vi "Create local tables from Server DB (old).vi"(8 "error in":errorcluster, 10 "Site":string="ICE1", 11 "tableNames":string[](array[string])) -> (0 "error out":errorcluster)   [LabVIEW 2010]
uses:
  <vilib>/addons/database/Auxilliary.llb/DB Tools DataTypes.ctl
  <vilib>/addons/database/Auxilliary.llb/DB Tools Cursor Type.ctl
  <vilib>/addons/database/_DB Variant To Data/Database Variant To Data.xnode
  <vilib>/addons/database/Connection.llb/DB Tools Open Connec (Path).vi
  <vilib>/addons/database/Connection.llb/Conn Execute.vi
  <vilib>/addons/database/Recordset.llb/Rec Fetch Recordset Data (R).vi
  <vilib>/addons/database/Recordset.llb/Rec Destroy - Connection.vi
  <vilib>/addons/database/NI_Database_API.lvlib
panel:
  out "column information":T2(array[cluster])
  out "columns":string[](array[string])
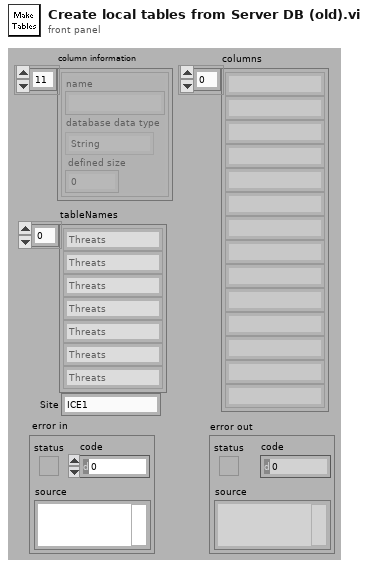
[diagram p1: front panel]
types:
  T1 = typedef "NI_Database_API.lvlib/DB Tools DataTypes.ctl" = enum16{"String", "Long (I32)", "Single (SGL)", "Double (DBL)", "Date/Time", "Binary"}
  T2 = cluster{"name":string, "database data type":T1, "defined size":i32}[]
  T3 = typedef "NI_Database_API.lvlib/DB Tools Cursor Type.ctl" = enum16{"forward-only", "keyset", "dynamic", "static"}
  T4 = typedef "NI_Database_API.lvlib/Conn ObjectReference.ctl" = refnum<k1>
  T5 = typedef "NI_Database_API.lvlib/Rec ObjectReference.ctl" = refnum<k1>
  T6 = cluster{"data":i32, "data":i32, "data":i32, "trimmed string":string, "trimmed string":string, "data":i32, "data":sgl, "data":i32, "data":i32, "data":i32, "trimmed string":string}
  T7 = cluster{"data":i32, "data":i32, "data":i32, "trimmed string":string, "data":i32, "data":i32, "trimmed string":string, "trimmed string":string, "trimmed string":string, "data":i32, "data":i32, "data":sgl, "data":i32, "data":i32, "trimmed string":string, "trimmed string":string}
  T8 = cluster{"data":i32, "trimmed string":string, "data":i32, "data":i32}
  T9 = cluster{"data":i32, "trimmed string":string, "data":i32, "trimmed string":string, "trimmed string":string, "trimmed string":string, "trimmed string":string, "data":sgl, "data":string, "trimmed string":string, "data":i32, "trimmed string":string, "trimmed string":string, "trimmed string":string}
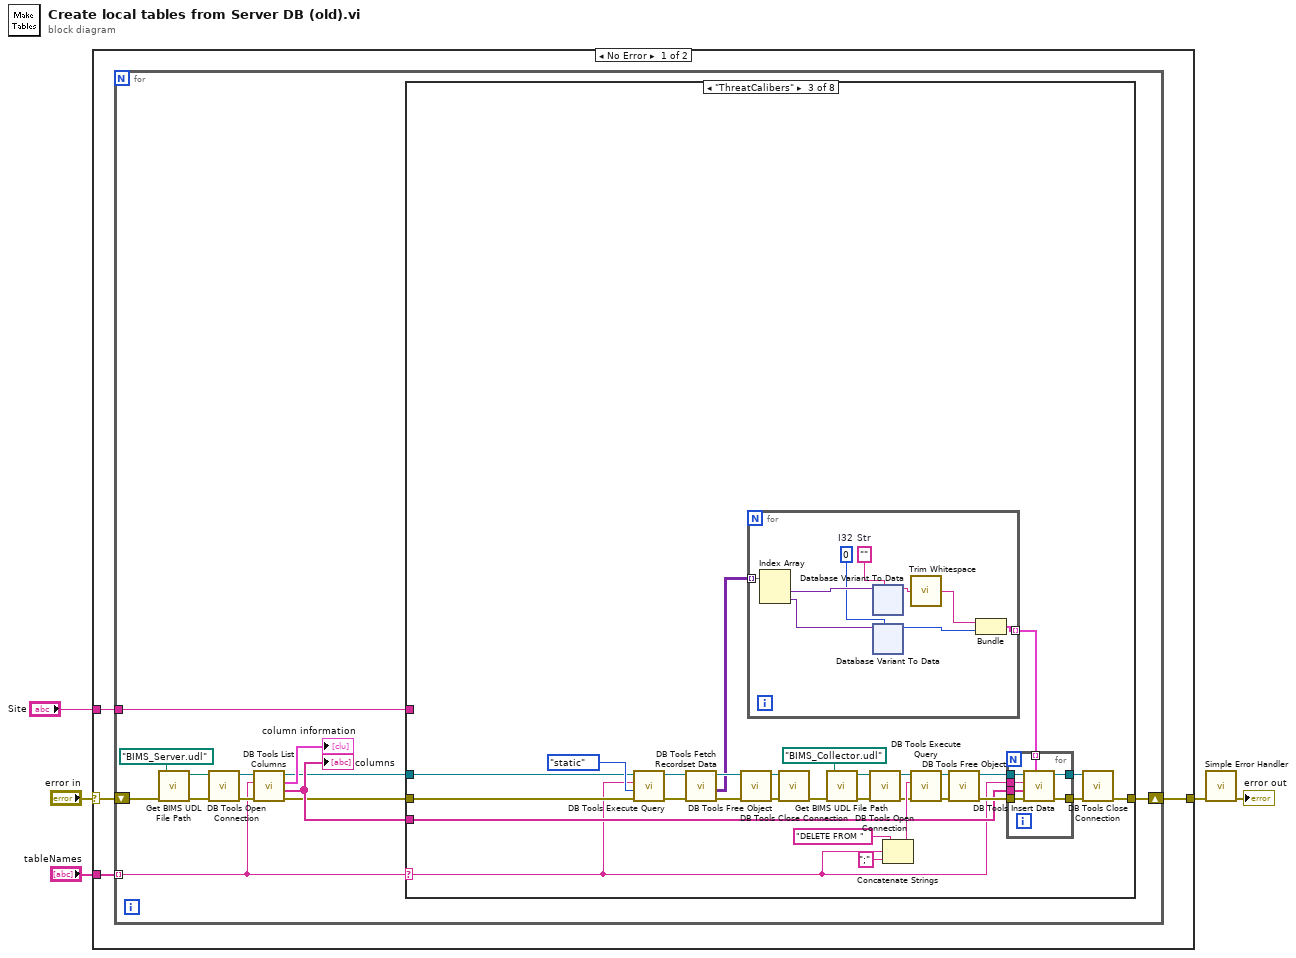
[diagram p0: block diagram]
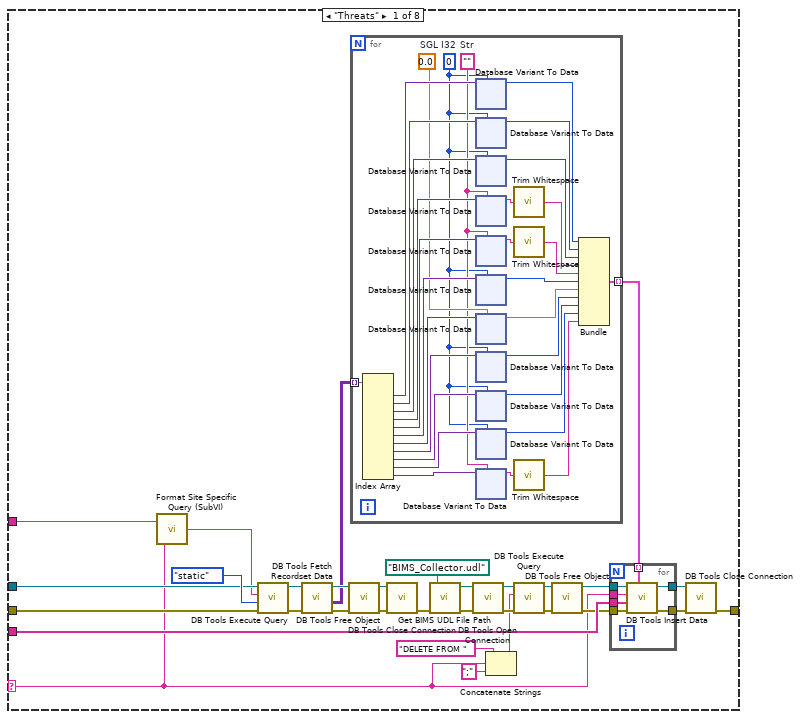
[diagram p2: hidden frame]
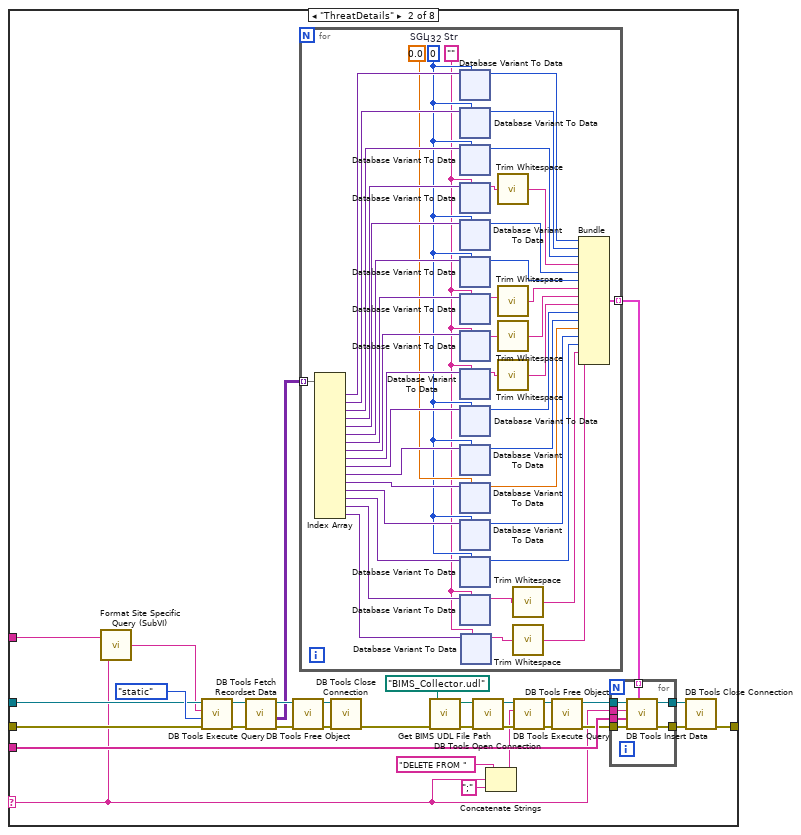
[diagram p3: hidden frame]
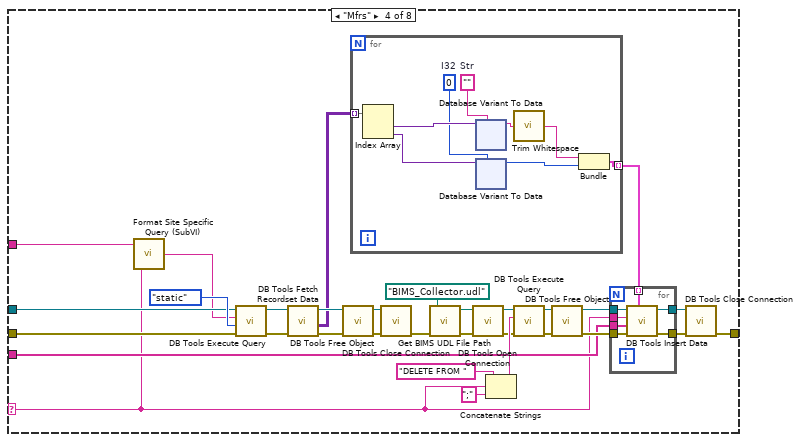
[diagram p4: hidden frame]
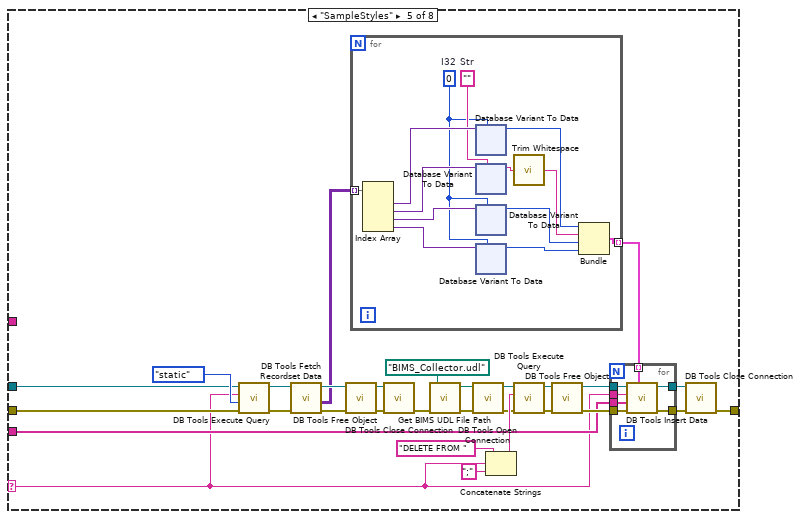
[diagram p5: hidden frame]
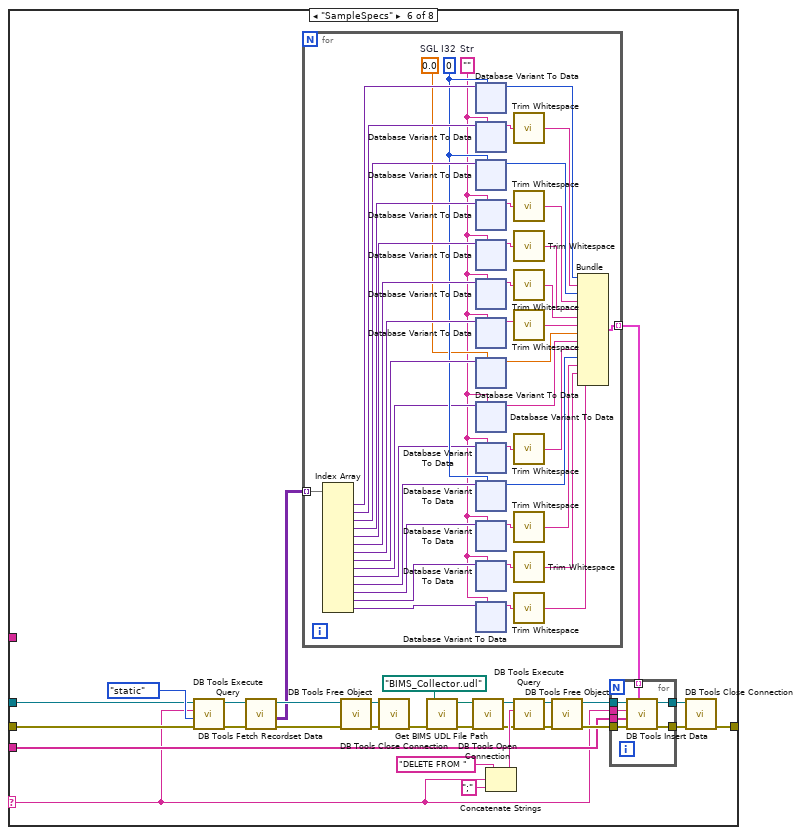
[diagram p6: hidden frame]
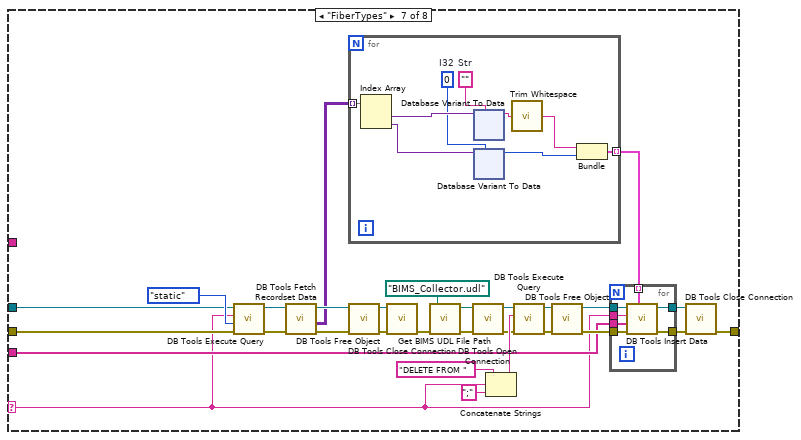
[diagram p7: hidden frame]
diagram:
  n1 = case shown="No Error" "error in" {
    selector: "error in" -> [w8 w2069]
    tunnel: [w9 w2069] -> w3
    tunnel: "tableNames" -> [w7 _]
    tunnel: "Site" -> [w6 _]
    frame No Error {
      n2 = for {
        tunnel: w7 -> [w16] mode=indexing
        shift-right: [w17] -> w9
        shift-left: w8 -> [w13]
        tunnel: w6 -> [w14]
        n3 = call "Get BIMS UDL File Path.vi"("error in"=w13, "UDL file name"=path "BIMS_Server.udl") -> ("error out"=w12:errorcluster, "Full UDL file path"=w21:path)  [unwired: 4 out]
        n4 = call-poly <vilib>:"DB Tools Open Connection.vi"("error in (no error)"=w12, "connection information"=w21) -> ("error out"=w20:errorcluster, "connection reference"=w11:T4)  [unwired: 3 in, 3 out]
        n5 = call <vilib>:"DB Tools List Columns.vi"("error in (no error)"=w20, "table"=w16, "connection reference"=w11) -> ("error out"=w15:errorcluster, "columns"=w18:string[], "column information"=→"column information":T2, "connection reference out"=w10:T4)  [unwired: 1 out]
        "columns" <- w18
        n6 = case shown="\"ThreatCalibers\"" w16 {
          selector: w16 -> [w25 w445 w1039 w1148 w1259 w1436 w1962 _]
          tunnel: w15 -> [w30 w450 w1041 w1152 w1261 w1438 w1963 w2068]
          tunnel: w18 -> [w51 w471 w1050 w1161 w1270 w1448 w1974 _]
          tunnel: [w38 w458 w1049 w1160 w1269 w1447 w1973 w2068] -> w17
          tunnel: w10 -> [w29 w449 w1040 w1151 w1258 w1437 w1961 _]
          tunnel: w14 -> [w26 w446 _ w1149 _ _ _ _]
          frame "Threats" {
            n7 = call "Format Site Specific Query (SubVI).vi"("Table"=w25, "Site"=w26) -> ("Query"=w27:string)
            n8 = call-poly <vilib>:"DB Tools Execute Query.vi"("error in (no error)"=w30, "cursor type"=DB_Tools_Cursor_Type."static", "SQL query"=w27, "connection reference"=w29) -> ("error out"=w36:errorcluster, "recordset reference"=w35:T5)  [unwired: 4 out]
            n9 = call-poly <vilib>:"DB Tools Fetch Recordset Data.vi"("error in (no error)"=w36, "recordset reference"=w35) -> ("error out"=w33:errorcluster, "recordset data"=w28:variant[][], "recordset reference out"=w34:T5)  [unwired: 3 out]
            n10 = call-poly <vilib>:"DB Tools Free Object.vi"("error in (no error)"=w33, "recordset reference"=w34) -> ("error out"=w31:errorcluster, "connection reference"=w32:T4)  [unwired: 8 out]
            n11 = for {
              tunnel: [w69] -> w48 mode=indexing
              tunnel: w28 -> [w90] mode=indexing
              w76 = sgl 0.0  # SGL
              w71 = ""  # Str
              w67 = 0  # I32
              n12 = Index Array(array=w90) -> (element #1=w89:variant, element #2=w88:variant, element #3=w85:variant, element #4=w84:variant, element #5=w83:variant, element #6=w82:variant, element #7=w81:variant, element #8=w80:variant, element #9=w75:variant, element #10=w73:variant, element #11=w70:variant)  [unwired: 11 in]
              n13 = xnode ("Database Variant To Data")("database variant"=w89, "type"=w67) -> ("data"=w68:i32)  [unwired: 1 in, 1 out]
              n14 = xnode "Database Variant To Data"("database variant"=w88, "type"=w67) -> ("data"=w87:i32)  [unwired: 1 in, 1 out]
              n15 = xnode "Database Variant To Data"("database variant"=w85, "type"=w67) -> ("data"=w86:i32)  [unwired: 1 in, 1 out]
              n16 = xnode "Database Variant To Data"("database variant"=w84, "type"=w71) -> ("data"=w66:string)  [unwired: 1 in, 1 out]
              n17 = xnode ("Database Variant To Data")("database variant"=w83, "type"=w71) -> ("data"=w64:string)  [unwired: 1 in, 1 out]
              n18 = xnode "Database Variant To Data"("database variant"=w82, "type"=w67) -> ("data"=w79:i32)  [unwired: 1 in, 1 out]
              n19 = xnode "Database Variant To Data"("database variant"=w81, "type"=w76) -> ("data"=w78:sgl)  [unwired: 1 in, 1 out]
              n20 = xnode "Database Variant To Data"("database variant"=w80, "type"=w67) -> ("data"=w77:i32)  [unwired: 1 in, 1 out]
              n21 = xnode "Database Variant To Data"("database variant"=w75, "type"=w67) -> ("data"=w74:i32)  [unwired: 1 in, 1 out]
              n22 = xnode "Database Variant To Data"("database variant"=w73, "type"=w67) -> ("data"=w72:i32)  [unwired: 1 in, 1 out]
              n23 = xnode "Database Variant To Data"("database variant"=w70, "type"=w71) -> ("data"=w62:string)  [unwired: 1 in, 1 out]
              n24 = call <vilib>:"Trim Whitespace.vi"("string"=w66) -> ("trimmed string"=w65:string)  [unwired: 1 in]
              n25 = call <vilib>:"Trim Whitespace.vi"("string"=w64) -> ("trimmed string"=w63:string)  [unwired: 1 in]
              n26 = call <vilib>:"Trim Whitespace.vi"("string"=w62) -> ("trimmed string"=w61:string)  [unwired: 1 in]
              n27 = Bundle("data"=w68, "data"=w87, "data"=w86, "trimmed string"=w65, "trimmed string"=w63, "data"=w79, "data"=w78, "data"=w77, "data"=w74, "data"=w72, "trimmed string"=w61) -> (w69:T6)  [unwired: 1 out]
            }
            n28 = call <vilib>:"DB Tools Close Connection.vi"("error in (no error)"=w31, "connection reference"=w32) -> ("error out"=w24:errorcluster)  [unwired: 5 out]
            n29 = call "Get BIMS UDL File Path.vi"("error in"=w24, "UDL file name"=path "BIMS_Collector.udl") -> ("error out"=w23:errorcluster, "Full UDL file path"=w53:path)  [unwired: 4 out]
            n30 = call-poly <vilib>:"DB Tools Open Connection.vi"("error in (no error)"=w23, "connection information"=w53) -> ("error out"=w47:errorcluster, "connection reference"=w44:T4)  [unwired: 3 in, 3 out]
            n31 = Concatenate Strings("DELETE FROM " ("SQL query"), w25, ";" ("string")) -> (w45:string)
            n32 = call-poly <vilib>:"DB Tools Execute Query.vi"("error in (no error)"=w47, "SQL query"=w45, "connection reference"=w44) -> ("error out"=w42:errorcluster, "recordset reference"=w40:T5)  [unwired: 1 in, 4 out]
            n33 = call-poly <vilib>:"DB Tools Free Object.vi"("error in (no error)"=w42, "recordset reference"=w40) -> ("error out"=w41:errorcluster, "connection reference"=w39:T4)  [unwired: 8 out]
            n34 = for {
              tunnel: [w60] -> w49
              tunnel: [w56] -> w50
              tunnel: w41 -> [w59]
              tunnel: w25 -> [w58]
              tunnel: w48 -> [w55] mode=indexing
              tunnel: w51 -> [w57]
              tunnel: w39 -> [w54]
              n35 = call <vilib>:"DB Tools Insert Data.vi"("data"=w55, "error in (no error)"=w59, "columns"=w57, "table"=w58, "connection reference"=w54) -> ("error out"=w56:errorcluster, "connection reference out"=w60:T4)  [unwired: 2 in, 3 out]
            }
            n36 = call <vilib>:"DB Tools Close Connection.vi"("error in (no error)"=w50, "connection reference"=w49) -> ("error out"=w38:errorcluster)  [unwired: 5 out]
          }
          frame "ThreatDetails" {
            n37 = call "Format Site Specific Query (SubVI).vi"("Table"=w445, "Site"=w446) -> ("Query"=w447:string)
            n38 = call-poly <vilib>:"DB Tools Execute Query.vi"("error in (no error)"=w450, "cursor type"=DB_Tools_Cursor_Type."static", "SQL query"=w447, "connection reference"=w449) -> ("error out"=w456:errorcluster, "recordset reference"=w455:T5)  [unwired: 4 out]
            n39 = call-poly <vilib>:"DB Tools Fetch Recordset Data.vi"("error in (no error)"=w456, "recordset reference"=w455) -> ("error out"=w453:errorcluster, "recordset data"=w448:variant[][], "recordset reference out"=w454:T5)  [unwired: 3 out]
            n40 = call-poly <vilib>:"DB Tools Free Object.vi"("error in (no error)"=w453, "recordset reference"=w454) -> ("error out"=w451:errorcluster, "connection reference"=w452:T4)  [unwired: 8 out]
            n41 = for {
              tunnel: [w507] -> w468 mode=indexing
              tunnel: w448 -> [w523] mode=indexing
              w494 = sgl 0.0  # SGL
              w483 = ""  # Str
              w490 = 0  # I32
              n42 = Index Array(array=w523) -> (element #1=w522:variant, element #2=w521:variant, element #3=w518:variant, element #4=w517:variant, element #5=w516:variant, element #6=w515:variant, element #7=w514:variant, element #8=w513:variant, element #9=w511:variant, element #10=w510:variant, element #11=w508:variant, element #12=w497:variant, element #13=w496:variant, element #14=w495:variant, element #15=w489:variant, element #16=w481:variant)  [unwired: 16 in]
              n43 = xnode ("Database Variant To Data")("database variant"=w522, "type"=w490) -> ("data"=w506:i32)  [unwired: 1 in, 1 out]
              n44 = xnode "Database Variant To Data"("database variant"=w521, "type"=w490) -> ("data"=w520:i32)  [unwired: 1 in, 1 out]
              n45 = xnode "Database Variant To Data"("database variant"=w518, "type"=w490) -> ("data"=w519:i32)  [unwired: 1 in, 1 out]
              n46 = xnode "Database Variant To Data"("database variant"=w517, "type"=w483) -> ("data"=w505:string)  [unwired: 1 in, 1 out]
              n47 = xnode ("Database Variant To Data")("database variant"=w516, "type"=w490) -> ("data"=w503:i32)  [unwired: 1 in, 1 out]
              n48 = xnode "Database Variant To Data"("database variant"=w515, "type"=w490) -> ("data"=w512:i32)  [unwired: 1 in, 1 out]
              n49 = xnode "Database Variant To Data"("database variant"=w514, "type"=w483) -> ("data"=w486:string)  [unwired: 1 in, 1 out]
              n50 = xnode "Database Variant To Data"("database variant"=w513, "type"=w483) -> ("data"=w502:string)  [unwired: 1 in, 1 out]
              n51 = xnode "Database Variant To Data"("database variant"=w511, "type"=w483) -> ("data"=w500:string)  [unwired: 1 in, 1 out]
              n52 = xnode "Database Variant To Data"("database variant"=w510, "type"=w490) -> ("data"=w509:i32)  [unwired: 1 in, 1 out]
              n53 = xnode "Database Variant To Data"("database variant"=w508, "type"=w490) -> ("data"=w498:i32)  [unwired: 1 in, 1 out]
              n54 = xnode "Database Variant To Data"("database variant"=w497, "type"=w494) -> ("data"=w493:sgl)  [unwired: 1 in, 1 out]
              n55 = xnode "Database Variant To Data"("database variant"=w496, "type"=w490) -> ("data"=w492:i32)  [unwired: 1 in, 1 out]
              n56 = xnode "Database Variant To Data"("database variant"=w495, "type"=w490) -> ("data"=w491:i32)  [unwired: 1 in, 1 out]
              n57 = xnode "Database Variant To Data"("database variant"=w489, "type"=w483) -> ("data"=w488:string)  [unwired: 1 in, 1 out]
              n58 = xnode "Database Variant To Data"("database variant"=w481, "type"=w483) -> ("data"=w484:string)  [unwired: 1 in, 1 out]
              n59 = call <vilib>:"Trim Whitespace.vi"("string"=w505) -> ("trimmed string"=w504:string)  [unwired: 1 in]
              n60 = call <vilib>:"Trim Whitespace.vi"("string"=w486) -> ("trimmed string"=w485:string)  [unwired: 1 in]
              n61 = call <vilib>:"Trim Whitespace.vi"("string"=w502) -> ("trimmed string"=w501:string)  [unwired: 1 in]
              n62 = call <vilib>:"Trim Whitespace.vi"("string"=w500) -> ("trimmed string"=w499:string)  [unwired: 1 in]
              n63 = call <vilib>:"Trim Whitespace.vi"("string"=w488) -> ("trimmed string"=w487:string)  [unwired: 1 in]
              n64 = call <vilib>:"Trim Whitespace.vi"("string"=w484) -> ("trimmed string"=w482:string)  [unwired: 1 in]
              n65 = Bundle("data"=w506, "data"=w520, "data"=w519, "trimmed string"=w504, "data"=w503, "data"=w512, "trimmed string"=w485, "trimmed string"=w501, "trimmed string"=w499, "data"=w509, "data"=w498, "data"=w493, "data"=w492, "data"=w491, "trimmed string"=w487, "trimmed string"=w482) -> (w507:T7)  [unwired: 1 out]
            }
            n66 = call <vilib>:"DB Tools Close Connection.vi"("error in (no error)"=w451, "connection reference"=w452) -> ("error out"=w444:errorcluster)  [unwired: 5 out]
            n67 = call "Get BIMS UDL File Path.vi"("error in"=w444, "UDL file name"=path "BIMS_Collector.udl") -> ("error out"=w443:errorcluster, "Full UDL file path"=w473:path)  [unwired: 4 out]
            n68 = call-poly <vilib>:"DB Tools Open Connection.vi"("error in (no error)"=w443, "connection information"=w473) -> ("error out"=w467:errorcluster, "connection reference"=w464:T4)  [unwired: 3 in, 3 out]
            n69 = Concatenate Strings("DELETE FROM " ("SQL query"), w445, ";" ("string")) -> (w465:string)
            n70 = call-poly <vilib>:"DB Tools Execute Query.vi"("error in (no error)"=w467, "SQL query"=w465, "connection reference"=w464) -> ("error out"=w462:errorcluster, "recordset reference"=w460:T5)  [unwired: 1 in, 4 out]
            n71 = call-poly <vilib>:"DB Tools Free Object.vi"("error in (no error)"=w462, "recordset reference"=w460) -> ("error out"=w461:errorcluster, "connection reference"=w459:T4)  [unwired: 8 out]
            n72 = for {
              tunnel: [w480] -> w469
              tunnel: [w476] -> w470
              tunnel: w461 -> [w479]
              tunnel: w445 -> [w478]
              tunnel: w468 -> [w475] mode=indexing
              tunnel: w471 -> [w477]
              tunnel: w459 -> [w474]
              n73 = call <vilib>:"DB Tools Insert Data.vi"("data"=w475, "error in (no error)"=w479, "columns"=w477, "table"=w478, "connection reference"=w474) -> ("error out"=w476:errorcluster, "connection reference out"=w480:T4)  [unwired: 2 in, 3 out]
            }
            n74 = call <vilib>:"DB Tools Close Connection.vi"("error in (no error)"=w470, "connection reference"=w469) -> ("error out"=w458:errorcluster)  [unwired: 5 out]
          }
          frame "ThreatCalibers" {
            n75 = call-poly <vilib>:"DB Tools Execute Query.vi"("error in (no error)"=w1041, "cursor type"=DB_Tools_Cursor_Type."static", "SQL query"=w1039, "connection reference"=w1040) -> ("error out"=w1045:errorcluster, "recordset reference"=w1044:T5)  [unwired: 4 out]
            n76 = call-poly <vilib>:"DB Tools Fetch Recordset Data.vi"("error in (no error)"=w1045, "recordset reference"=w1044) -> ("error out"=w1046:errorcluster, "recordset data"=w1038:variant[][], "recordset reference out"=w1043:T5)  [unwired: 3 out]
            n77 = call-poly <vilib>:"DB Tools Free Object.vi"("error in (no error)"=w1046, "recordset reference"=w1043) -> ("error out"=w1047:errorcluster, "connection reference"=w1042:T4)  [unwired: 8 out]
            n78 = for {
              tunnel: [w1076] -> w1055 mode=indexing
              tunnel: w1038 -> [w1080] mode=indexing
              w1072 = ""  # Str
              w1073 = 0  # I32
              n79 = Index Array(array=w1080) -> (element #1=w1079:variant, element #2=w1078:variant)  [unwired: 2 in]
              n80 = xnode ("Database Variant To Data")("database variant"=w1079, "type"=w1072) -> ("data"=w1075:string)  [unwired: 1 in, 1 out]
              n81 = xnode "Database Variant To Data"("database variant"=w1078, "type"=w1073) -> ("data"=w1077:i32)  [unwired: 1 in, 1 out]
              n82 = call <vilib>:"Trim Whitespace.vi"("string"=w1075) -> ("trimmed string"=w1074:string)  [unwired: 1 in]
              n83 = Bundle("trimmed string"=w1074, "data"=w1077) -> (w1076:cluster{"trimmed string":string, "data":i32})  [unwired: 1 out]
            }
            n84 = call <vilib>:"DB Tools Close Connection.vi"("error in (no error)"=w1047, "connection reference"=w1042) -> ("error out"=w1037:errorcluster)  [unwired: 5 out]
            n85 = call "Get BIMS UDL File Path.vi"("error in"=w1037, "UDL file name"=path "BIMS_Collector.udl") -> ("error out"=w1036:errorcluster, "Full UDL file path"=w1051:path)  [unwired: 4 out]
            n86 = call-poly <vilib>:"DB Tools Open Connection.vi"("error in (no error)"=w1036, "connection information"=w1051) -> ("error out"=w1056:errorcluster, "connection reference"=w1059:T4)  [unwired: 3 in, 3 out]
            n87 = Concatenate Strings("DELETE FROM " ("SQL query"), w1039, ";" ("string")) -> (w1058:string)
            n88 = call-poly <vilib>:"DB Tools Execute Query.vi"("error in (no error)"=w1056, "SQL query"=w1058, "connection reference"=w1059) -> ("error out"=w1061:errorcluster, "recordset reference"=w1063:T5)  [unwired: 1 in, 4 out]
            n89 = call-poly <vilib>:"DB Tools Free Object.vi"("error in (no error)"=w1061, "recordset reference"=w1063) -> ("error out"=w1062:errorcluster, "connection reference"=w1064:T4)  [unwired: 8 out]
            n90 = for {
              tunnel: [w1071] -> w1054
              tunnel: [w1067] -> w1053
              tunnel: w1062 -> [w1070]
              tunnel: w1039 -> [w1069]
              tunnel: w1055 -> [w1066] mode=indexing
              tunnel: w1050 -> [w1068]
              tunnel: w1064 -> [w1065]
              n91 = call <vilib>:"DB Tools Insert Data.vi"("data"=w1066, "error in (no error)"=w1070, "columns"=w1068, "table"=w1069, "connection reference"=w1065) -> ("error out"=w1067:errorcluster, "connection reference out"=w1071:T4)  [unwired: 2 in, 3 out]
            }
            n92 = call <vilib>:"DB Tools Close Connection.vi"("error in (no error)"=w1053, "connection reference"=w1054) -> ("error out"=w1049:errorcluster)  [unwired: 5 out]
          }
          frame "Mfrs" {
            n93 = call "Format Site Specific Query (SubVI).vi"("Table"=w1148, "Site"=w1149) -> ("Query"=w1147:string)
            n94 = call-poly <vilib>:"DB Tools Execute Query.vi"("error in (no error)"=w1152, "cursor type"=DB_Tools_Cursor_Type."static", "SQL query"=w1147, "connection reference"=w1151) -> ("error out"=w1156:errorcluster, "recordset reference"=w1155:T5)  [unwired: 4 out]
            n95 = call-poly <vilib>:"DB Tools Fetch Recordset Data.vi"("error in (no error)"=w1156, "recordset reference"=w1155) -> ("error out"=w1157:errorcluster, "recordset data"=w1150:variant[][], "recordset reference out"=w1154:T5)  [unwired: 3 out]
            n96 = call-poly <vilib>:"DB Tools Free Object.vi"("error in (no error)"=w1157, "recordset reference"=w1154) -> ("error out"=w1158:errorcluster, "connection reference"=w1153:T4)  [unwired: 8 out]
            n97 = for {
              tunnel: [w1189] -> w1166 mode=indexing
              tunnel: w1150 -> [w1191] mode=indexing
              w1186 = ""  # Str
              w1185 = 0  # I32
              n98 = Index Array(array=w1191) -> (element #1=w1187:variant, element #2=w1190:variant)  [unwired: 2 in]
              n99 = xnode "Database Variant To Data"("database variant"=w1187, "type"=w1186) -> ("data"=w1184:string)  [unwired: 1 in, 1 out]
              n100 = xnode ("Database Variant To Data")("database variant"=w1190, "type"=w1185) -> ("data"=w1183:i32)  [unwired: 1 in, 1 out]
              n101 = call <vilib>:"Trim Whitespace.vi"("string"=w1184) -> ("trimmed string"=w1188:string)  [unwired: 1 in]
              n102 = Bundle("trimmed string"=w1188, "data"=w1183) -> (w1189:cluster{"trimmed string":string, "data":i32})  [unwired: 1 out]
            }
            n103 = call <vilib>:"DB Tools Close Connection.vi"("error in (no error)"=w1158, "connection reference"=w1153) -> ("error out"=w1146:errorcluster)  [unwired: 5 out]
            n104 = call "Get BIMS UDL File Path.vi"("error in"=w1146, "UDL file name"=path "BIMS_Collector.udl") -> ("error out"=w1145:errorcluster, "Full UDL file path"=w1162:path)  [unwired: 4 out]
            n105 = call-poly <vilib>:"DB Tools Open Connection.vi"("error in (no error)"=w1145, "connection information"=w1162) -> ("error out"=w1167:errorcluster, "connection reference"=w1170:T4)  [unwired: 3 in, 3 out]
            n106 = Concatenate Strings("DELETE FROM " ("SQL query"), w1148, ";" ("string")) -> (w1169:string)
            n107 = call-poly <vilib>:"DB Tools Execute Query.vi"("error in (no error)"=w1167, "SQL query"=w1169, "connection reference"=w1170) -> ("error out"=w1172:errorcluster, "recordset reference"=w1174:T5)  [unwired: 1 in, 4 out]
            n108 = call-poly <vilib>:"DB Tools Free Object.vi"("error in (no error)"=w1172, "recordset reference"=w1174) -> ("error out"=w1173:errorcluster, "connection reference"=w1175:T4)  [unwired: 8 out]
            n109 = for {
              tunnel: [w1182] -> w1165
              tunnel: [w1178] -> w1164
              tunnel: w1173 -> [w1181]
              tunnel: w1148 -> [w1180]
              tunnel: w1166 -> [w1177] mode=indexing
              tunnel: w1161 -> [w1179]
              tunnel: w1175 -> [w1176]
              n110 = call <vilib>:"DB Tools Insert Data.vi"("data"=w1177, "error in (no error)"=w1181, "columns"=w1179, "table"=w1180, "connection reference"=w1176) -> ("error out"=w1178:errorcluster, "connection reference out"=w1182:T4)  [unwired: 2 in, 3 out]
            }
            n111 = call <vilib>:"DB Tools Close Connection.vi"("error in (no error)"=w1164, "connection reference"=w1165) -> ("error out"=w1160:errorcluster)  [unwired: 5 out]
          }
          frame "SampleStyles" {
            n112 = call-poly <vilib>:"DB Tools Execute Query.vi"("error in (no error)"=w1261, "cursor type"=DB_Tools_Cursor_Type."static", "SQL query"=w1259, "connection reference"=w1258) -> ("error out"=w1265:errorcluster, "recordset reference"=w1264:T5)  [unwired: 4 out]
            n113 = call-poly <vilib>:"DB Tools Fetch Recordset Data.vi"("error in (no error)"=w1265, "recordset reference"=w1264) -> ("error out"=w1266:errorcluster, "recordset data"=w1260:variant[][], "recordset reference out"=w1263:T5)  [unwired: 3 out]
            n114 = call-poly <vilib>:"DB Tools Free Object.vi"("error in (no error)"=w1266, "recordset reference"=w1263) -> ("error out"=w1267:errorcluster, "connection reference"=w1262:T4)  [unwired: 8 out]
            n115 = for {
              tunnel: [w1300] -> w1275 mode=indexing
              tunnel: w1260 -> [w1304] mode=indexing
              w1296 = ""  # Str
              w1295 = 0  # I32
              n116 = Index Array(array=w1304) -> (element #1=w1297:variant, element #2=w1298:variant, element #3=w1303:variant, element #4=w1302:variant)  [unwired: 4 in]
              n117 = xnode ("Database Variant To Data")("database variant"=w1297, "type"=w1295) -> ("data"=w1293:i32)  [unwired: 1 in, 1 out]
              n118 = xnode "Database Variant To Data"("database variant"=w1298, "type"=w1296) -> ("data"=w1294:string)  [unwired: 1 in, 1 out]
              n119 = xnode ("Database Variant To Data")("database variant"=w1303, "type"=w1295) -> ("data"=w1292:i32)  [unwired: 1 in, 1 out]
              n120 = xnode "Database Variant To Data"("database variant"=w1302, "type"=w1295) -> ("data"=w1301:i32)  [unwired: 1 in, 1 out]
              n121 = call <vilib>:"Trim Whitespace.vi"("string"=w1294) -> ("trimmed string"=w1299:string)  [unwired: 1 in]
              n122 = Bundle("data"=w1293, "trimmed string"=w1299, "data"=w1292, "data"=w1301) -> (w1300:T8)  [unwired: 1 out]
            }
            n123 = call <vilib>:"DB Tools Close Connection.vi"("error in (no error)"=w1267, "connection reference"=w1262) -> ("error out"=w1257:errorcluster)  [unwired: 5 out]
            n124 = call "Get BIMS UDL File Path.vi"("error in"=w1257, "UDL file name"=path "BIMS_Collector.udl") -> ("error out"=w1256:errorcluster, "Full UDL file path"=w1271:path)  [unwired: 4 out]
            n125 = call-poly <vilib>:"DB Tools Open Connection.vi"("error in (no error)"=w1256, "connection information"=w1271) -> ("error out"=w1276:errorcluster, "connection reference"=w1279:T4)  [unwired: 3 in, 3 out]
            n126 = Concatenate Strings("DELETE FROM " ("SQL query"), w1259, ";" ("string")) -> (w1278:string)
            n127 = call-poly <vilib>:"DB Tools Execute Query.vi"("error in (no error)"=w1276, "SQL query"=w1278, "connection reference"=w1279) -> ("error out"=w1281:errorcluster, "recordset reference"=w1283:T5)  [unwired: 1 in, 4 out]
            n128 = call-poly <vilib>:"DB Tools Free Object.vi"("error in (no error)"=w1281, "recordset reference"=w1283) -> ("error out"=w1282:errorcluster, "connection reference"=w1284:T4)  [unwired: 8 out]
            n129 = for {
              tunnel: [w1291] -> w1274
              tunnel: [w1287] -> w1273
              tunnel: w1282 -> [w1290]
              tunnel: w1259 -> [w1289]
              tunnel: w1275 -> [w1286] mode=indexing
              tunnel: w1270 -> [w1288]
              tunnel: w1284 -> [w1285]
              n130 = call <vilib>:"DB Tools Insert Data.vi"("data"=w1286, "error in (no error)"=w1290, "columns"=w1288, "table"=w1289, "connection reference"=w1285) -> ("error out"=w1287:errorcluster, "connection reference out"=w1291:T4)  [unwired: 2 in, 3 out]
            }
            n131 = call <vilib>:"DB Tools Close Connection.vi"("error in (no error)"=w1273, "connection reference"=w1274) -> ("error out"=w1269:errorcluster)  [unwired: 5 out]
          }
          frame "SampleSpecs" {
            n132 = call-poly <vilib>:"DB Tools Execute Query.vi"("error in (no error)"=w1438, "cursor type"=DB_Tools_Cursor_Type."static", "SQL query"=w1436, "connection reference"=w1437) -> ("error out"=w1442:errorcluster, "recordset reference"=w1441:T5)  [unwired: 4 out]
            n133 = call-poly <vilib>:"DB Tools Fetch Recordset Data.vi"("error in (no error)"=w1442, "recordset reference"=w1441) -> ("error out"=w1443:errorcluster, "recordset data"=w1435:variant[][], "recordset reference out"=w1440:T5)  [unwired: 3 out]
            n134 = for {
              tunnel: [w1491] -> w1446 mode=indexing
              tunnel: w1435 -> [w1503] mode=indexing
              w1466 = sgl 0.0  # SGL
              w1463 = ""  # Str
              w1489 = 0  # I32
              n135 = Index Array(array=w1503) -> (element #1=w1502:variant, element #2=w1501:variant, element #3=w1499:variant, element #4=w1498:variant, element #5=w1497:variant, element #6=w1496:variant, element #7=w1495:variant, element #8=w1494:variant, element #9=w1467:variant, element #10=w1468:variant, element #11=w1469:variant, element #12=w1470:variant, element #13=w1471:variant, element #14=w1464:variant)  [unwired: 14 in]
              n136 = xnode ("Database Variant To Data")("database variant"=w1502, "type"=w1489) -> ("data"=w1490:i32)  [unwired: 1 in, 1 out]
              n137 = xnode "Database Variant To Data"("database variant"=w1501, "type"=w1463) -> ("data"=w1482:string)  [unwired: 1 in, 1 out]
              n138 = xnode "Database Variant To Data"("database variant"=w1499, "type"=w1489) -> ("data"=w1500:i32)  [unwired: 1 in, 1 out]
              n139 = xnode "Database Variant To Data"("database variant"=w1498, "type"=w1463) -> ("data"=w1488:string)  [unwired: 1 in, 1 out]
              n140 = xnode ("Database Variant To Data")("database variant"=w1497, "type"=w1463) -> ("data"=w1486:string)  [unwired: 1 in, 1 out]
              n141 = xnode "Database Variant To Data"("database variant"=w1496, "type"=w1463) -> ("data"=w1476:string)  [unwired: 1 in, 1 out]
              n142 = xnode "Database Variant To Data"("database variant"=w1495, "type"=w1463) -> ("data"=w1478:string)  [unwired: 1 in, 1 out]
              n143 = xnode "Database Variant To Data"("database variant"=w1494, "type"=w1466) -> ("data"=w1493:sgl)  [unwired: 1 in, 1 out]
              n144 = xnode "Database Variant To Data"("database variant"=w1467, "type"=w1463) -> ("data"=w1472:string)  [unwired: 1 in, 1 out]
              n145 = xnode "Database Variant To Data"("database variant"=w1468, "type"=w1463) -> ("data"=w1480:string)  [unwired: 1 in, 1 out]
              n146 = xnode "Database Variant To Data"("database variant"=w1469, "type"=w1489) -> ("data"=w1492:i32)  [unwired: 1 in, 1 out]
              n147 = xnode "Database Variant To Data"("database variant"=w1470, "type"=w1463) -> ("data"=w1484:string)  [unwired: 1 in, 1 out]
              n148 = xnode "Database Variant To Data"("database variant"=w1471, "type"=w1463) -> ("data"=w1474:string)  [unwired: 1 in, 1 out]
              n149 = xnode "Database Variant To Data"("database variant"=w1464, "type"=w1463) -> ("data"=w1465:string)  [unwired: 1 in, 1 out]
              n150 = call <vilib>:"Trim Whitespace.vi"("string"=w1482) -> ("trimmed string"=w1481:string)  [unwired: 1 in]
              n151 = call <vilib>:"Trim Whitespace.vi"("string"=w1488) -> ("trimmed string"=w1487:string)  [unwired: 1 in]
              n152 = call <vilib>:"Trim Whitespace.vi"("string"=w1486) -> ("trimmed string"=w1485:string)  [unwired: 1 in]
              n153 = call <vilib>:"Trim Whitespace.vi"("string"=w1476) -> ("trimmed string"=w1475:string)  [unwired: 1 in]
              n154 = call <vilib>:"Trim Whitespace.vi"("string"=w1478) -> ("trimmed string"=w1477:string)  [unwired: 1 in]
              n155 = call <vilib>:"Trim Whitespace.vi"("string"=w1480) -> ("trimmed string"=w1479:string)  [unwired: 1 in]
              n156 = call <vilib>:"Trim Whitespace.vi"("string"=w1484) -> ("trimmed string"=w1483:string)  [unwired: 1 in]
              n157 = call <vilib>:"Trim Whitespace.vi"("string"=w1474) -> ("trimmed string"=w1473:string)  [unwired: 1 in]
              n158 = call <vilib>:"Trim Whitespace.vi"("string"=w1465) -> ("trimmed string"=w1462:string)  [unwired: 1 in]
              n159 = Bundle("data"=w1490, "trimmed string"=w1481, "data"=w1500, "trimmed string"=w1487, "trimmed string"=w1485, "trimmed string"=w1475, "trimmed string"=w1477, "data"=w1493, "data"=w1472, "trimmed string"=w1479, "data"=w1492, "trimmed string"=w1483, "trimmed string"=w1473, "trimmed string"=w1462) -> (w1491:T9)  [unwired: 1 out]
            }
            n160 = call-poly <vilib>:"DB Tools Free Object.vi"("error in (no error)"=w1443, "recordset reference"=w1440) -> ("error out"=w1444:errorcluster, "connection reference"=w1439:T4)  [unwired: 8 out]
            n161 = call <vilib>:"DB Tools Close Connection.vi"("error in (no error)"=w1444, "connection reference"=w1439) -> ("error out"=w1434:errorcluster)  [unwired: 5 out]
            n162 = call "Get BIMS UDL File Path.vi"("error in"=w1434, "UDL file name"=path "BIMS_Collector.udl") -> ("error out"=w1433:errorcluster, "Full UDL file path"=w1449:path)  [unwired: 4 out]
            n163 = call-poly <vilib>:"DB Tools Open Connection.vi"("error in (no error)"=w1433, "connection information"=w1449) -> ("error out"=w1453:errorcluster, "connection reference"=w1456:T4)  [unwired: 3 in, 3 out]
            n164 = Concatenate Strings("DELETE FROM " ("SQL query"), w1436, ";" ("string")) -> (w1455:string)
            n165 = call-poly <vilib>:"DB Tools Execute Query.vi"("error in (no error)"=w1453, "SQL query"=w1455, "connection reference"=w1456) -> ("error out"=w1458:errorcluster, "recordset reference"=w1460:T5)  [unwired: 1 in, 4 out]
            n166 = call-poly <vilib>:"DB Tools Free Object.vi"("error in (no error)"=w1458, "recordset reference"=w1460) -> ("error out"=w1459:errorcluster, "connection reference"=w1461:T4)  [unwired: 8 out]
            n167 = for {
              tunnel: [w1958] -> w1452
              tunnel: [w1954] -> w1451
              tunnel: w1459 -> [w1957]
              tunnel: w1436 -> [w1956]
              tunnel: w1446 -> [w1953] mode=indexing
              tunnel: w1448 -> [w1955]
              tunnel: w1461 -> [w1952]
              n168 = call <vilib>:"DB Tools Insert Data.vi"("data"=w1953, "error in (no error)"=w1957, "columns"=w1955, "table"=w1956, "connection reference"=w1952) -> ("error out"=w1954:errorcluster, "connection reference out"=w1958:T4)  [unwired: 2 in, 3 out]
            }
            n169 = call <vilib>:"DB Tools Close Connection.vi"("error in (no error)"=w1451, "connection reference"=w1452) -> ("error out"=w1447:errorcluster)  [unwired: 5 out]
          }
          frame "FiberTypes" {
            n170 = call-poly <vilib>:"DB Tools Execute Query.vi"("error in (no error)"=w1963, "cursor type"=DB_Tools_Cursor_Type."static", "SQL query"=w1962, "connection reference"=w1961) -> ("error out"=w1970:errorcluster, "recordset reference"=w1969:T5)  [unwired: 4 out]
            n171 = call-poly <vilib>:"DB Tools Fetch Recordset Data.vi"("error in (no error)"=w1970, "recordset reference"=w1969) -> ("error out"=w1967:errorcluster, "recordset data"=w1964:variant[][], "recordset reference out"=w1968:T5)  [unwired: 3 out]
            n172 = for {
              tunnel: [w1992] -> w1972 mode=indexing
              tunnel: w1964 -> [w1996] mode=indexing
              w1988 = ""  # Str
              w1989 = 0  # I32
              n173 = Index Array(array=w1996) -> (element #1=w1995:variant, element #2=w1994:variant)  [unwired: 2 in]
              n174 = xnode ("Database Variant To Data")("database variant"=w1995, "type"=w1988) -> ("data"=w1991:string)  [unwired: 1 in, 1 out]
              n175 = xnode "Database Variant To Data"("database variant"=w1994, "type"=w1989) -> ("data"=w1993:i32)  [unwired: 1 in, 1 out]
              n176 = call <vilib>:"Trim Whitespace.vi"("string"=w1991) -> ("trimmed string"=w1990:string)  [unwired: 1 in]
              n177 = Bundle("trimmed string"=w1990, "data"=w1993) -> (w1992:cluster{"trimmed string":string, "data":i32})  [unwired: 1 out]
            }
            n178 = call-poly <vilib>:"DB Tools Free Object.vi"("error in (no error)"=w1967, "recordset reference"=w1968) -> ("error out"=w1965:errorcluster, "connection reference"=w1966:T4)  [unwired: 8 out]
            n179 = call <vilib>:"DB Tools Close Connection.vi"("error in (no error)"=w1965, "connection reference"=w1966) -> ("error out"=w1960:errorcluster)  [unwired: 5 out]
            n180 = call "Get BIMS UDL File Path.vi"("error in"=w1960, "UDL file name"=path "BIMS_Collector.udl") -> ("error out"=w1959:errorcluster, "Full UDL file path"=w1975:path)  [unwired: 4 out]
            n181 = call-poly <vilib>:"DB Tools Open Connection.vi"("error in (no error)"=w1959, "connection information"=w1975) -> ("error out"=w1979:errorcluster, "connection reference"=w1982:T4)  [unwired: 3 in, 3 out]
            n182 = Concatenate Strings("DELETE FROM " ("SQL query"), w1962, ";" ("string")) -> (w1981:string)
            n183 = call-poly <vilib>:"DB Tools Execute Query.vi"("error in (no error)"=w1979, "SQL query"=w1981, "connection reference"=w1982) -> ("error out"=w1984:errorcluster, "recordset reference"=w1986:T5)  [unwired: 1 in, 4 out]
            n184 = call-poly <vilib>:"DB Tools Free Object.vi"("error in (no error)"=w1984, "recordset reference"=w1986) -> ("error out"=w1985:errorcluster, "connection reference"=w1987:T4)  [unwired: 8 out]
            n185 = for {
              tunnel: [w2067] -> w1978
              tunnel: [w2063] -> w1977
              tunnel: w1985 -> [w2066]
              tunnel: w1962 -> [w2065]
              tunnel: w1972 -> [w2062] mode=indexing
              tunnel: w1974 -> [w2064]
              tunnel: w1987 -> [w2061]
              n186 = call <vilib>:"DB Tools Insert Data.vi"("data"=w2062, "error in (no error)"=w2066, "columns"=w2064, "table"=w2065, "connection reference"=w2061) -> ("error out"=w2063:errorcluster, "connection reference out"=w2067:T4)  [unwired: 2 in, 3 out]
            }
            n187 = call <vilib>:"DB Tools Close Connection.vi"("error in (no error)"=w1977, "connection reference"=w1978) -> ("error out"=w1973:errorcluster)  [unwired: 5 out]
          }
          frame "Information", Default {
            # "The following case has a structure determined for \n  the Threats table in the BIMS server.\n\n  The data retieved from the table is site specific."
          }
        }
      }
    }
    frame Error {
    }
  }
  n188 = call <vilib>:"Simple Error Handler.vi"("error in (no error)"=w3) -> ("error out"=→"error out":errorcluster)  [unwired: 1 in, 7 out]
